vi "ConfigureServo.vi"(8 "error in":errorcluster, 10 "ServoConfiguration":T1={"Servo Max Steps"=10, "Servo Min Steps"=2, "Servo Initial Averaging Time (s)"=0.0001, "Servo Final Averaging Time (s)"=0.0004, "Servo Active Servo Window (s)"=0.001, "Servo Tolerance (dB)"=0.05} {"Servo Active Servo Window (s)" format="%#_6e"; "Servo Final Averaging Time (s)" format="%#_6p"; "Servo Initial Averaging Time (s)" format="%#_6p"}, 11 "ServoSessionIn":u32) -> (0 "error out":errorcluster, 3 "ServoSessionOut":u32)   [LabVIEW 2016, in "Power Servo.lvlib"]
uses:
  Power Servo.lvlib
  Type Definitions/Servo Configuration.ctl
  Type Definitions/RFSA Reference Trigger Override.ctl
  Type Definitions/Enable.ctl
  <userlib>/_NI Power Servoing IP/HostRdl/NI Power Servoing IP New (Host).lvlib
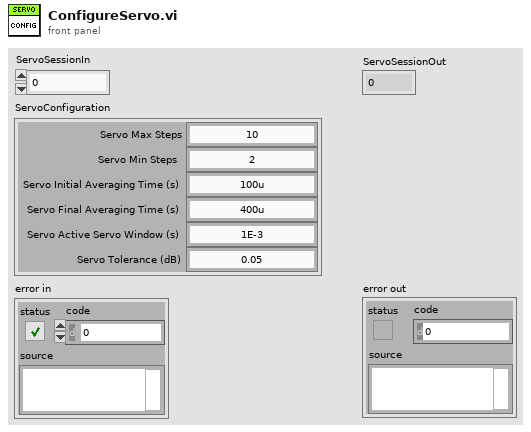
[diagram p1: front panel]
types:
  T1 = typedef "Power Servo.lvlib/Servo Configuration.ctl" = cluster{"Servo Max Steps":u16, "Servo Min Steps":u16, "Servo Initial Averaging Time (s)":dbl, "Servo Final Averaging Time (s)":dbl, "Servo Active Servo Window (s)":dbl, "Servo Tolerance (dB)":dbl}
  T2 = typedef "Power Servo.lvlib/Enable.ctl" = enum16{"False", "True"}
  T3 = typedef "Power Servo.lvlib/RFSA Reference Trigger Override.ctl" = u16
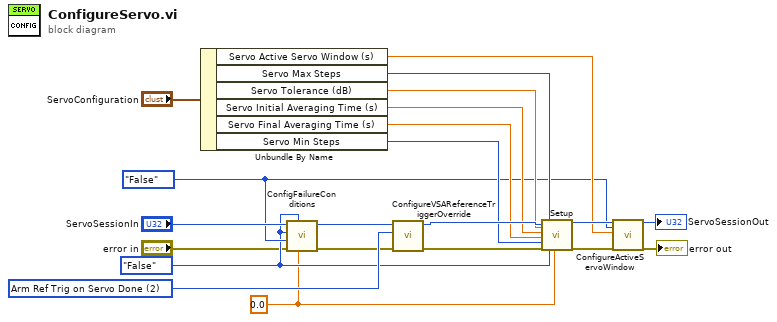
[diagram p0: block diagram]
diagram:
  w3 = 0.0 ("ContinuousStepSize")
  w4 = Enable."False" ("Enable")
  w20 = T3 2 items=["Immediate  Ref Trig on Servo Done"=1, "Arm Ref Trig on Servo Done"=2] ("RFSA Reference Trigger Override")
  w5 = Enable."False" ("Enable")
  n1 = Unbundle By Name("ServoConfiguration") -> ("Servo Active Servo Window (s)"=w10:dbl, "Servo Max Steps"=w17:u16, "Servo Tolerance (dB)"=w16:dbl, "Servo Initial Averaging Time (s)"=w15:dbl, "Servo Final Averaging Time (s)"=w14:dbl, "Servo Min Steps"=w13:u16)
  n2 = call <userlib>:"ConfigFailureConditions.vi"("servo_failure_cfg_disable_saturation_threshold"=w3, "servo_failure_cfg_disable_fail_on_saturation"=w4, "error in"="error in", "servo_failure_cfg_disable_reset_on_fail"=w5, "servo_failure_cfg_disable_gain_step_limit"=w4, "SessionHandleIn"="ServoSessionIn") -> ("error out"=w2:errorcluster, "SessionHandleOut"=w6:u32)  [unwired: 4 in]
  n3 = call <userlib>:"ConfigureVSAReferenceTriggerOverride.vi"("error in"=w2, "RefTrigOverride"=w20, "SessionHandleIn"=w6) -> ("error out"=w18:errorcluster, "SessionHandleOut"=w19:u32)  [unwired: 7 in]
  n4 = call <userlib>:"Setup.vi"("SessionHandleIn"=w19, "DesiredAccuracyDB"=w16, "InitialAveragingTimeS"=w15, "FinalAveragingTimeS"=w14, "MinumumNumberOfAverages"=w13, "error in"=w18, "NumStepsUntilError"=w17, "continuous"=w4, "ContinuousStepSize"=w3) -> ("SessionHandleOut"=w12:u32, "error out"=w11:errorcluster)  [unwired: 9 in]
  n5 = call <userlib>:"ConfigureActiveServoWindow.vi"("SessionHandleIn"=w12, "ActiveWindowEnabled"=w5, "ActiveWindowLengthS"=w10, "error in"=w11) -> ("SessionHandleOut"=→"ServoSessionOut":u32, "error out"=→"error out":errorcluster)  [unwired: 14 in]
